vi "Read Leaf.vi"(7 "Actor in":refnum<class "Actor.lvclass">) -> (2 "Leaf":bool)   [LabVIEW 2020, in "jettl.lvlib" / "Actor Specific.lvlib"]
uses:
  Actor Specific.lvlib
  Actor/Actor.lvclass
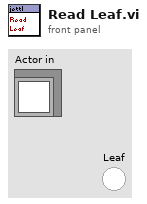
[diagram p1: front panel]
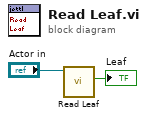
[diagram p0: block diagram]
diagram:
  n1 = call-dynamic "Read Leaf.vi"("Actor in"="Actor in") -> ("Leaf"=→"Leaf":bool)  [unwired: 10 in]
